vi "csv_path_from_binary.vi"(10 "extension":string=".csv", 11 "path to binary file":path) -> (3 "path to spec. ext.":path)   [LabVIEW 2017]
uses:
  <vilib>/regexp/Match Regular Expression.xnode
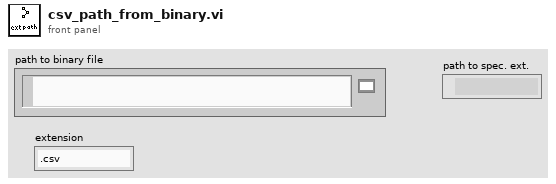
[diagram p1: front panel]
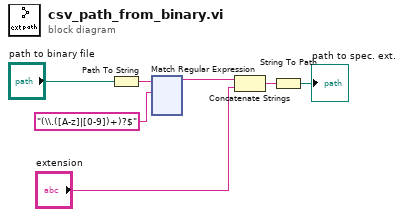
[diagram p0: block diagram]
diagram:
  n1 = Path To String(path="path to binary file") -> (string=w4:string)
  n2 = xnode "Match Regular Expression"("input string"=w4, "regular expression"="(\\.([A-z]|[0-9])+)?$") -> ("before match"=w7:string)  [unwired: 4 in, 4 out]
  n3 = Concatenate Strings(w7, "extension") -> (w5:string)
  n4 = String To Path(string=w5) -> (path=→"path to spec. ext.":path)
